vi "Add Library and Class Hierarchy Levels.vi"(11 "Hierarchy Array":string[](array[string])) -> (3 "Modified Hierarchy Array":string[](array[string]))   [LabVIEW 2023]
doc: "Modifies <B>Hierarchy Array</B> based on the presence of .lvlib or .lvclass files, and current LabVIEW folder hierarchy standards for those items."
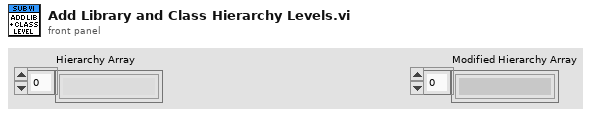
[diagram p1: front panel]
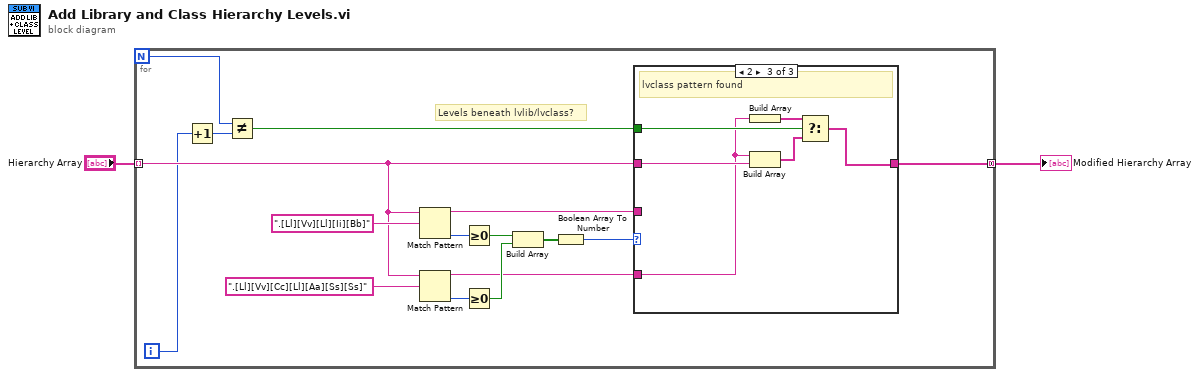
[diagram p0: block diagram]
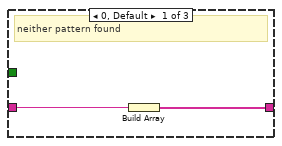
[diagram p2: hidden frame]
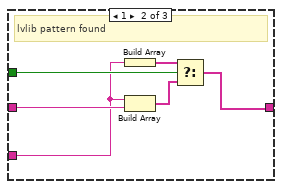
[diagram p3: hidden frame]
diagram:
  n1 = for {
    N -> [w4]
    tunnel: "Hierarchy Array" -> [w10] mode=indexing
    tunnel: [w9] -> w1 mode=concatenating
    i -> [w6]
    # "Levels beneath lvlib/lvclass?"
    n2 = Increment(x=w6) -> (x+1=w5:i32)
    n3 = Not Equal?(x=w4, y=w5) -> (x != y?=w3:bool)
    n4 = Match Pattern(string=w10, regular expression=".[Ll][Vv][Ll][Ii][Bb]" ("search string/char (-)")) -> (before substring=w8:string, offset past match=w16:i32)  [unwired: 1 in, 2 out]
    n5 = Match Pattern(string=w10, regular expression=".[Ll][Vv][Cc][Ll][Aa][Ss][Ss]" ("search string/char (-)")) -> (before substring=w7:string, offset past match=w15:i32)  [unwired: 1 in, 2 out]
    n6 = Greater Or Equal To 0?(x=w16) -> (x >= 0?=w14:bool)
    n7 = Greater Or Equal To 0?(x=w15) -> (x >= 0?=w13:bool)
    n8 = Build Array(w14, w13) -> (w12:bool[])
    n9 = Boolean Array To Number(Boolean array=w12) -> (number=w11:u32)
    n10 = case shown="2" w11 {
      tunnel: w10 -> [w20 w26 w32]
      tunnel: [w19 w21 w28] -> w9
      tunnel: w8 -> [_ w23 _]
      tunnel: w7 -> [_ _ w27]
      tunnel: w3 -> [_ w25 w31]
      frame 0, Default {
        # "neither pattern found"
        n11 = Build Array(w20) -> (w19:string[])
      }
      frame 1 {
        # "lvlib pattern found"
        n12 = Build Array(w23) -> (w22:string[])
        n13 = Build Array(w23, w26) -> (w24:string[])
        n14 = Select(t=w22, s=w25, f=w24) -> (s? t:f=w21:string[])
      }
      frame 2 {
        # "lvclass pattern found"
        n15 = Build Array(w27) -> (w29:string[])
        n16 = Build Array(w27, w32) -> (w30:string[])
        n17 = Select(t=w29, s=w31, f=w30) -> (s? t:f=w28:string[])
      }
    }
  }
  "Modified Hierarchy Array" <- w1
